vi "ExTestCCDdim2.vi"() -> ()   [LabVIEW 2010]
panel:
  out "after init y dimension":u32
  out "after init x dimension":u32
  out "Y dimension":u32
  out "Y dimension programed":u32
  out "X dimension":u32
  out "X dimension programed":u32
  out "error out":errorcluster
  in  "error in (no error)":errorcluster
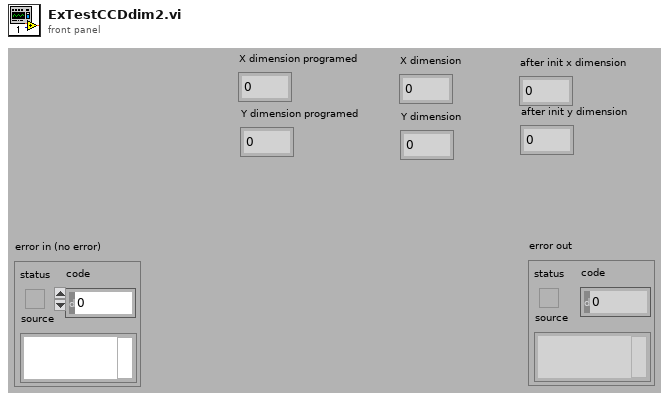
[diagram p1: front panel]
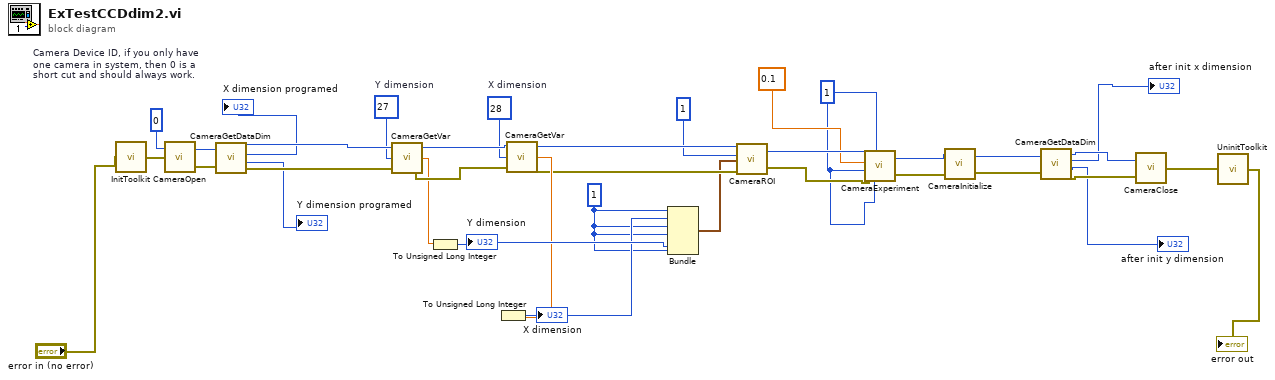
[diagram p0: block diagram]
diagram:
  w8 = 1
  w10 = 1
  w24 = 28  # X dimension
  w25 = 27  # Y dimension
  w35 = 0  # Camera Device ID, if you only have  one camera in system, then 0 is a  short cut and should always work.
  n1 = call <userlib>:"InitToolkit.vi"("error in"="error in (no error)") -> ("error out"=w36:errorcluster)
  n2 = call <userlib>:"CameraOpen.vi"("error in"=w36, "Camera Device ID"=w35) -> ("error out"=w31:errorcluster, "Camera Handle"=w30:u32)
  n3 = call <userlib>:"CameraGetDataDim.vi"("Camera Handle"=w30, "error in"=w31) -> ("Camera Handle"=w29:u32, "Xdim"=→"X dimension programed":u32, "Ydim"=→"Y dimension programed":u32, "error out"=w28:errorcluster)
  n4 = call <userlib>:"CameraGetVar.vi"("error in"=w28, "Parameter ID"=w25, "Camera Handle"=w29) -> ("error out"=w27:errorcluster, "Value"=w18:dbl, "Camera Handle"=w26:u32)
  n5 = To Unsigned Long Integer(number=w18) -> (unsigned 32bit integer=w21:u32)
  "Y dimension" <- w21
  n6 = call <userlib>:"CameraGetVar.vi"("error in"=w27, "Parameter ID"=w24, "Camera Handle"=w26) -> ("error out"=w14:errorcluster, "Value"=w19:dbl, "Camera Handle"=w13:u32)
  n7 = To Unsigned Long Integer(number=w19) -> (unsigned 32bit integer=w20:u32)
  "X dimension" <- w20
  n8 = Bundle(w8, w20, w8, w8, w21, w8) -> (w7:cluster{i32, u32, i32, i32, u32, i32})  [unwired: 1 in]
  n9 = call <userlib>:"CameraROI.vi"("error in"=w14, "ROI Params"=w7, "ROI Index"=1, "Camera Handle"=w13) -> ("error out"=w17:errorcluster, "Camera Handle"=w12:u32)
  n10 = call <userlib>:"CameraExperiment.vi"("Number of Accumulations"=w10, "Acquire / Focus Flag"=w10, "error in"=w17, "Number of Images"=w10, "Exposure (sec)"=0.1, "Camera Handle"=w12) -> ("error out"=w16:errorcluster, "Camera Handle"=w15:u32)
  n11 = call <userlib>:"CameraInitialize.vi"("error in"=w16, "Camera Handle"=w15) -> ("error out"=w6:errorcluster, "Camera Handle"=w4:u32)
  n12 = call <userlib>:"CameraGetDataDim.vi"("Camera Handle"=w4, "error in"=w6) -> ("Camera Handle"=w3:u32, "Xdim"=→"after init x dimension":u32, "Ydim"=→"after init y dimension":u32, "error out"=w5:errorcluster)
  n13 = call <userlib>:"CameraClose.vi"("error in"=w5, "Camera Handle"=w3) -> ("error out"=w32:errorcluster)
  n14 = call <userlib>:"UninitToolkit.vi"("error in"=w32) -> ("error out"=→"error out":errorcluster)
